vi "extract_exe_archive.vi"(8 "error in (no error)":errorcluster, 9 "preview?":bool, 10 "archive_path":path, 11 "target_path in":path) -> (0 "error out":errorcluster, 1 "files []":path[](array[path]), 2 "archive_path out":path, 3 "target_path out":path)   [LabVIEW 2015, in "lv-bin-7zip.lvlib" / "v1.lvlib"]
uses:
  v1.lvlib
  lv-bin-7zip.lvlib
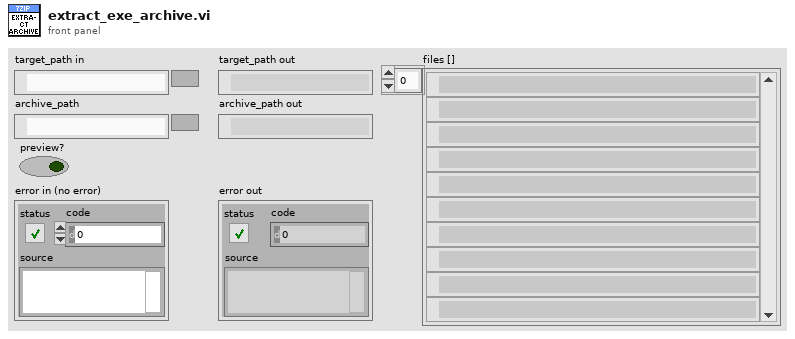
[diagram p1: front panel]
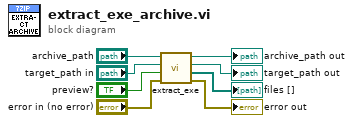
[diagram p0: block diagram]
diagram:
  n1 = call "extract_exe.vi"("error in (no error)"="error in (no error)", "preview?"="preview?", "target_path in"="target_path in", "archive_path (file_dialog)"="archive_path") -> ("error out"=→"error out":errorcluster, "files []"=→"files []":path[], "target_path out"=→"target_path out":path, "archive_path out"=→"archive_path out":path)  [unwired: 4 in]
